vi "Release.vi"(8 "error in (no error)":errorcluster, 11 "Queue in":refnum<queue>) -> (0 "error out":errorcluster, 2 "Remaining Elements":string[](array[string]), 3 "Queue Name":string)   [LabVIEW 2021, in "Queue.lvlib"]
doc: "Force release a queue reference and remove the named queue from the cache if exists. Obtaining named queues do not need to be released. The same reference is returned each time.\n\n<b>Warning: Releasing a queue always force destroys the queue reference.</b>"
uses:
  Queue.lvlib
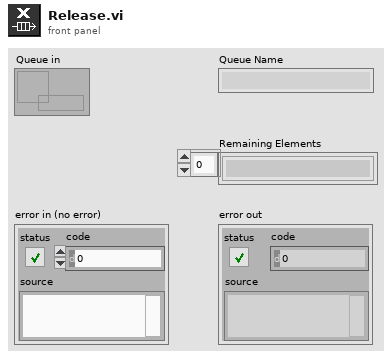
[diagram p1: front panel]
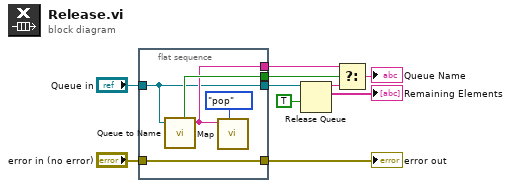
[diagram p0: block diagram]
diagram:
  n1 = flat-sequence {
    tunnel: "Queue in" -> [w12]
    tunnel: [w14] -> w7
    tunnel: [w13] -> w5
    tunnel: [w12] -> w4
    tunnel: [w11] -> w2
    tunnel: "error in (no error)" -> [w11]
    frame #0 {
      n2 = call "Queue to Name.vi"("Queue in"=w12) -> ("Found?"=w14:bool, "Queue Name out"=w13:string)  [unwired: 7 in]
      n3 = call "Map.vi"("Action"=enum8{"noop", "get", "set", "pop"}."pop", "Queue Name"=w13) -> ()  [unwired: 7 in, 3 out]
    }
  }
  n4 = Release Queue(queue=w4, force destroy? (F)=TRUE ("Force Destroy? (T)")) -> (queue name=w6:string, remaining elements=→"Remaining Elements":string[])  [unwired: 1 in, 1 out]
  n5 = Select(t=w5, s=w7, f=w6) -> (s? t:f=→"Queue Name":string)
  "error out" <- w2
